vi "Event Msg To Self.vi"(10 "Msg":refnum<class "Msg.lvclass">, 11 "Ex Event Actor in":refnum<class "Ex Event Actor.lvclass">) -> (0 "error out":errorcluster)   [LabVIEW 2021, in "Ex Event Actor.lvlib" / "Ex Event Actor.lvclass"]
uses:
  Ex Event Actor.lvclass
  Ex Event Actor.lvclass/Ex Event Actor.ctl
  Actor/Event Actor/Event Actor.lvclass
  Actor/Msg/Msg.lvclass
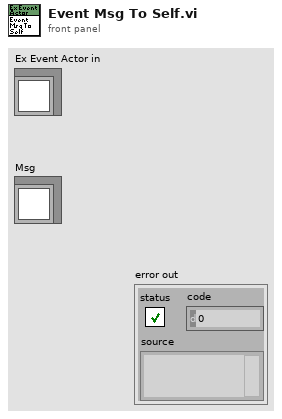
[diagram p1: front panel]
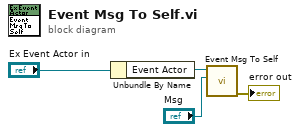
[diagram p0: block diagram]
diagram:
  n1 = Unbundle By Name("Ex Event Actor in") -> ("Event Actor"=w3:refnum<class "Event Actor.lvclass">)
  n2 = call-dynamic "Event Msg To Self.vi"("Msg"="Msg", "Event Actor in"=w3) -> ("error out"=→"error out":errorcluster)  [unwired: 9 in]
